vi "Rot_Key_Freq.vi"(11 "Rotation":dbl) -> (2 "Key Position":u8, 3 "Fundamental Frequency":dbl)   [LabVIEW 2016]
uses:
  <vilib>/express/express arith-compare/Formula/XNode/ExpressFormulaBlockNode.xnode
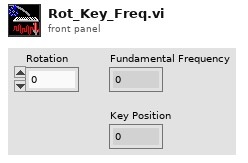
[diagram p1: front panel]
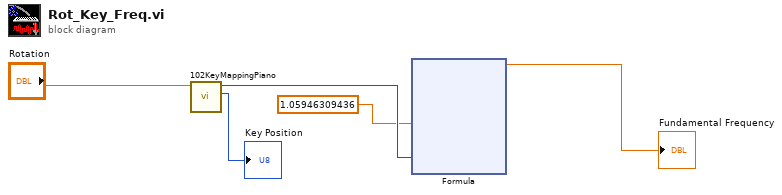
[diagram p0: block diagram]
diagram:
  n1 = call "102KeyMappingPiano.vi"("Double"="Rotation") -> ("signed 8bit integer"=→"Key Position":u8, "Numeric"=w2:i8)  [unwired: 9 in]
  n2 = xnode "Formula"("X1"=1.05946309436, "X2"=w2) -> ("Result"=→"Fundamental Frequency":dbl)  [unwired: 1 in, 1 out]
